vi "Calc_subvi.vi"() -> ()   [LabVIEW 2018]
panel:
  in  "열거형":T1(ring)
  in  "A":dbl
  in  "B":dbl
  out "Operator":string
  out "Result":dbl
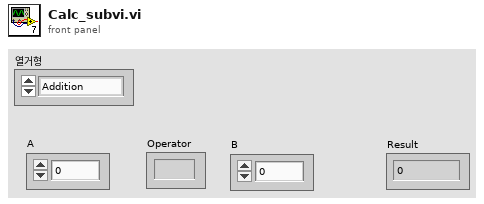
[diagram p1: front panel]
types:
  T1 = enum16{"Addition", "Subtract", "Division", "Multiply"}
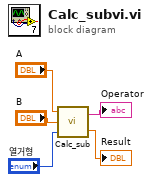
[diagram p0: block diagram]
diagram:
  n1 = call "Calc_sub.vi"("열거형"="열거형", "B"="B", "A"="A") -> ("숫자형 컨트롤"=→"Result":dbl, "문자열"=→"Operator":string)  [unwired: 1 in]
